vi "JX_SetHomePosition_SubVI.vi"(8 "error in (no error)":errorcluster, 10 "channel":i32, 11 "MB Serial Master:MB_Master":refnum<class "MB_Master.lvclass">) -> (0 "error out":errorcluster, 2 "Registers":u16[](array[numeric]), 3 "MB Serial Master:MB_Master":refnum<class "MB_Master.lvclass">)   [LabVIEW 2023, in "Jiaxin_Stepper_Controller.lvlib"]
uses:
  Jiaxin_Stepper_Controller.lvlib
  <vilib>/Plasmionique/MB Master/MB_Master/MB_Master.lvclass
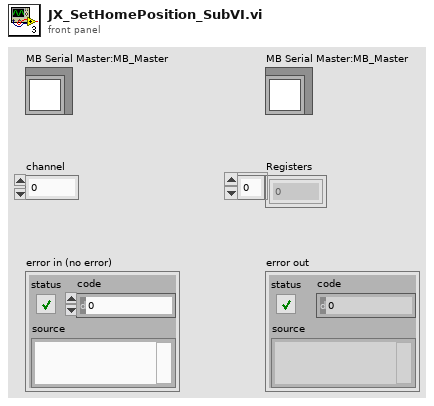
[diagram p1: front panel]
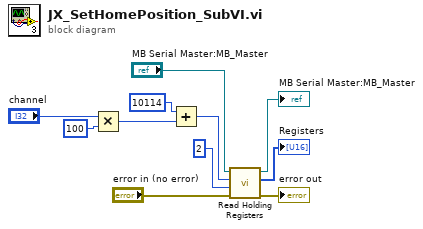
[diagram p0: block diagram]
diagram:
  n1 = Multiply(x="channel", y=100) -> (x*y=w6:i32)
  n2 = Add(x=10114, y=w6) -> (x+y=w5:i32)
  n3 = call <vilib>:"Read Holding Registers.vi"("error in (no error)"="error in (no error)", "quantity"=u16 2, "starting address"=w5, "MB session in"="MB Serial Master:MB_Master") -> ("error out"=→"error out":errorcluster, "Registers"=→"Registers":u16[], "MB session out"=→"MB Serial Master:MB_Master":refnum<class "MB_Master.lvclass">)  [unwired: 5 in]
